vi "symmetric_from_upper_triangle.vi"(10 "Data":dbl[](array[numeric]), 11 "Size":i32) -> (3 "Array out":dbl[][](array[numeric]))   [LabVIEW 2012]
panel:
  # "Create a symmetrical (square) array from flat upper triangle data."
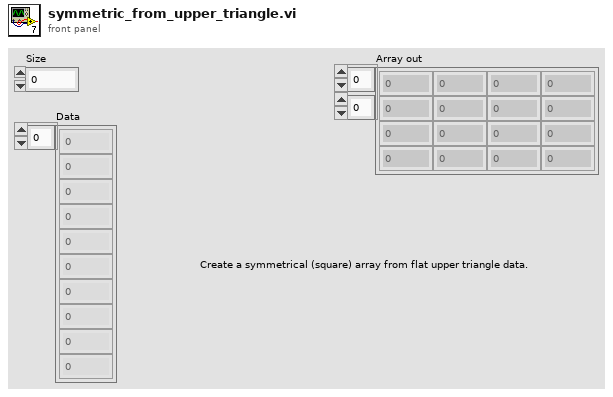
[diagram p1: front panel]
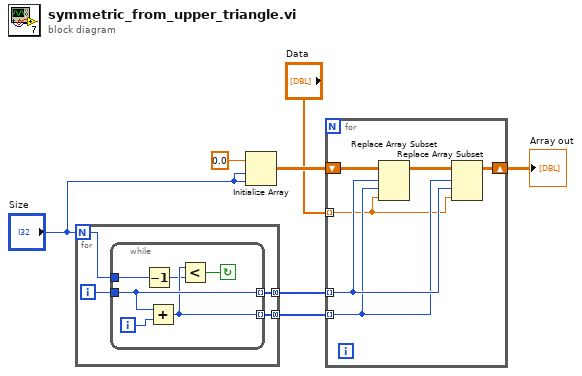
[diagram p0: block diagram]
diagram:
  n1 = for {
    N: "Size" -> [w11]
    tunnel: [w9] -> w2 mode=concatenating
    tunnel: [w8] -> w1 mode=concatenating
    i -> [w10]
    n2 = while {
      tunnel: w10 -> [w15]
      tunnel: w11 -> [w12]
      tunnel: [w14] -> w9 mode=indexing
      tunnel: [w15] -> w8 mode=indexing
      i -> [w17]
      stop <- w16 continue-if-true
      n3 = Decrement(x=w12) -> (x-1=w13:i32)
      n4 = Add(x=w15, y=w17) -> (x+y=w14:i32)
      n5 = Less?(x=w14, y=w13) -> (x < y?=w16:bool)
    }
  }
  n6 = Initialize Array(0.0 ("element"), "Size", "Size") -> (w6:dbl[][])
  n7 = for {
    tunnel: w2 -> [w21] mode=indexing
    tunnel: "Data" -> [w20] mode=indexing
    tunnel: w1 -> [w22] mode=indexing
    shift-right: [w18] -> w7
    shift-left: w6 -> [w23]
    n8 = Replace Array Subset(array=w23, new element=w20, index (row)=w22, index (col)=w21) -> (w19:dbl[][])
    n9 = Replace Array Subset(array=w19, new element=w20, index (row)=w21, index (col)=w22) -> (w18:dbl[][])
  }
  "Array out" <- w7
